vi "NumIntegrate_Rkf45_Func_A.vi"(9 "Col":i32, 11 "Row":i32) -> (3 "RKF45_A":dbl)   [LabVIEW 2019, in "Trajectory_Library.lvlib"]
doc: "Internal function used by Rkdp_Impl.vi\n\nInputs:\n - Row -- Row to look up ( 0 - 4 )\n - Column -- Column value to look up ( 0 - 4 )\n\nOutputs:\n - A -- Value looked up by index."
uses:
  Trajectory_Library.lvlib
  <vilib>/Analysis/Matrix/Datatypes/RealMatrix.ctl
  <vilib>/Analysis/Matrix/NI_Matrix.lvlib
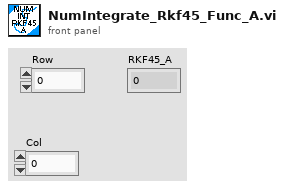
[diagram p1: front panel]
types:
  T1 = typedef "NI_Matrix.lvlib/RealMatrix.ctl" = dbl[][]
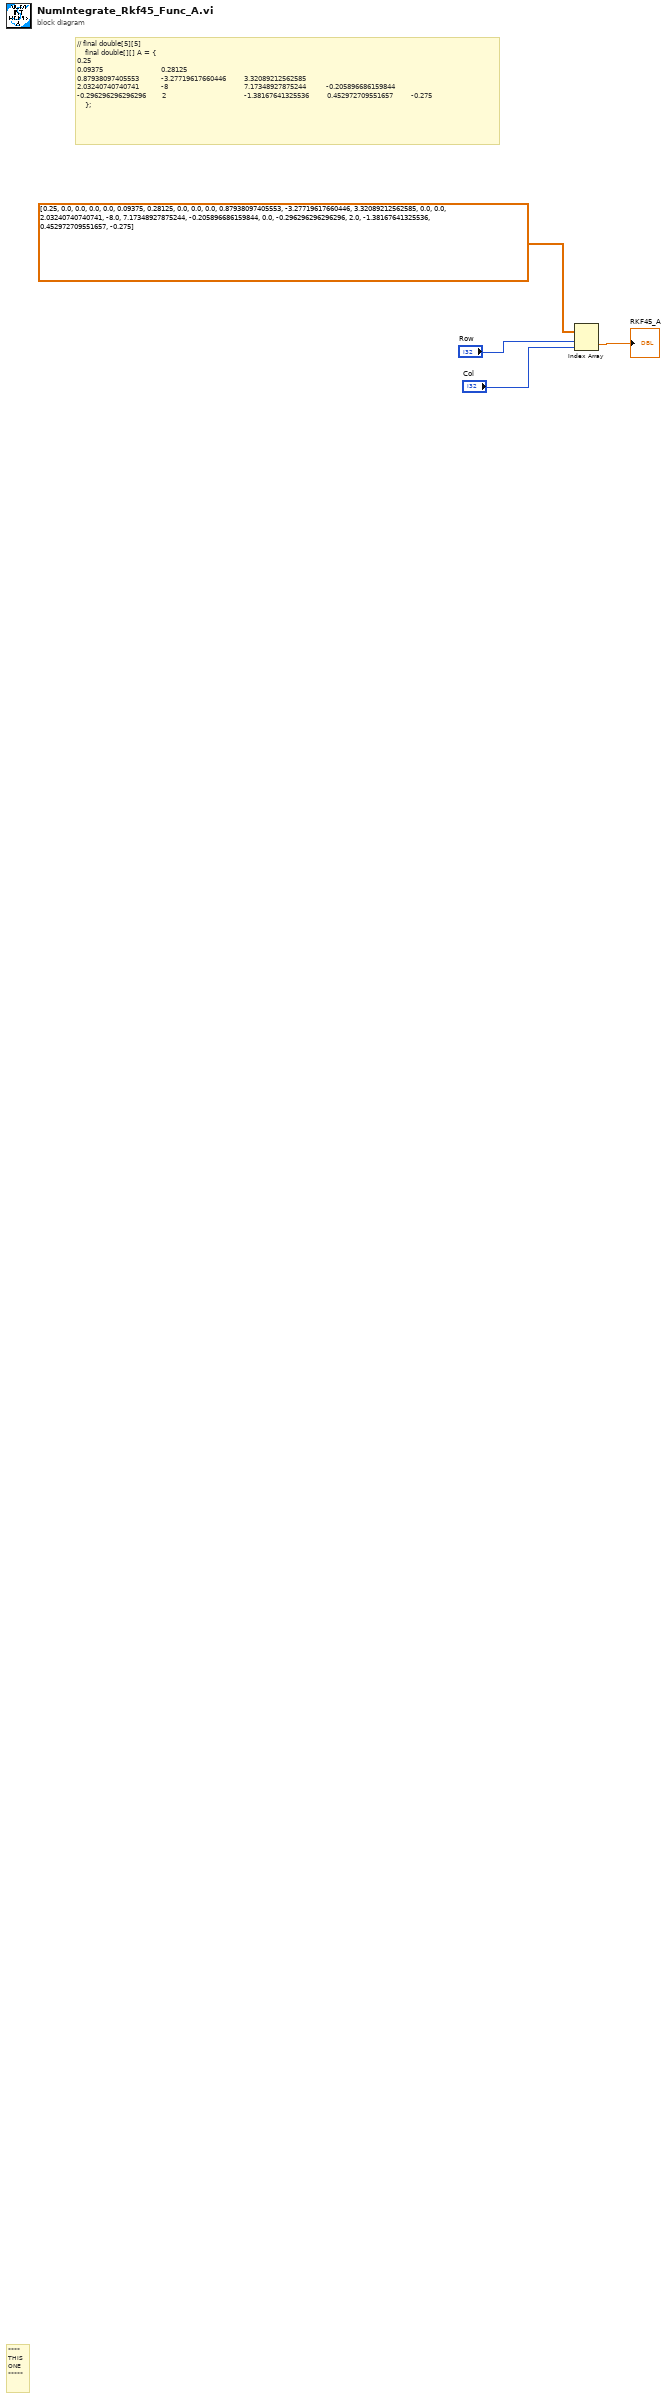
[diagram p0: block diagram]
diagram:
  # "// final double[5][5]\t\t\t\t\n    final double[][] A = {\t\t\t\t\n0.25\t\t\t\t\n0.09375\t                            0.28125\t\t\t\n0.87938097405553   \t       -3.27719617660446\t        3.32089212562585\t\t\n2.03240740740741\t          -8\t                                     7.17348927875244  \t       -0.205896686159844\t\n-0.296296296296296\t       2\t                                      -1.38167641325536\t        0.452972709551657\t        -0.275\n    };"
  # "****\nTHIS\nONE\n*****"
  n1 = Index Array(array=T1 [[0.25, 0.0, 0.0, 0.0, 0.0], [0.09375, 0.28125, 0.0, 0.0, 0.0], [0.87938097405553, -3.27719617660446, 3.32089212562585, 0.0, 0.0], [2.03240740740741, -8.0, 7.17348927875244, -0.205896686159844, 0.0], [-0.296296296296296, 2.0, -1.38167641325536, 0.452972709551657, -0.275]] ("matrix"), index (row)="Row", index (col)="Col") -> (element=→"RKF45_A":dbl)
